vi "DAQmx Create Channel (Power).vi"(0 "task in":refnum<k21>, 1 "voltage setpoint":dbl, 2 "current setpoint":dbl=0.03, 5 "physical channels":tag, 7 "name to assign":string, 9 "output enable":bool=TRUE, 11 "error in":errorcluster) -> (4 "task out":refnum<k21>, 15 "error out":errorcluster)   [LabVIEW 2024]
doc: "Creates channel(s) to source and measure power."
uses:
  nilvaiu.dll
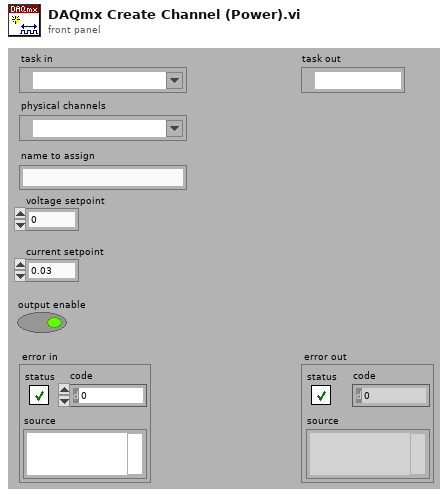
[diagram p1: front panel]
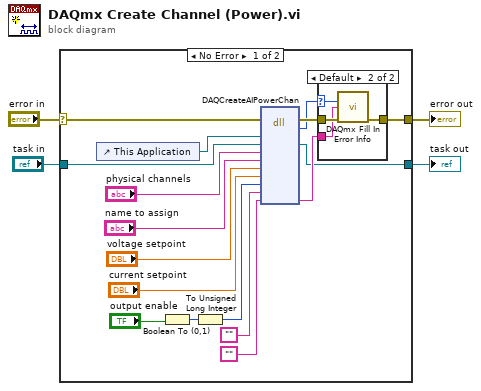
[diagram p0: block diagram]
diagram:
  n1 = case shown="No Error" "error in" {
    selector: "error in" -> [w17 w28]
    tunnel: [w16 w28] -> w4
    tunnel: [w15 w27] -> w3
    tunnel: "task in" -> [w14 w27]
    frame No Error {
      n2 = control-ref of="This Application"() -> (w18:refnum<vi>)
      n3 = Boolean To (0,1)(Boolean="output enable") -> (0, 1=w7:i16)
      n4 = To Unsigned Long Integer(number=w7) -> (unsigned 32bit integer=w5:u32)
      n5 = dll-call lib="nilvaiu.*" fn="DAQCreateAIPowerChan"(error in=w17, "lvAppRef"=w18, "refObjPtr"=w14, "physicalChannelName"="physical channels", "channelNameIn"="name to assign", "voltageSetpoint"="voltage setpoint", "currentSetpoint"="current setpoint", "OutputEnable"=w5, "channelNamesOut"="", "extendedErrorInfo"="") -> (error out=w21:errorcluster, "return type"=w20:i32, "refObjPtr"=w15:refnum<k21>, "extendedErrorInfo"=w19:string)  [unwired: 9 in, 1 out]
      n6 = case shown="Default" w20 {
        selector: w20 -> [_ w24]
        tunnel: w21 -> [w22 w26]
        tunnel: [w22 w25] -> w16
        tunnel: w19 -> [_ w23]
        frame 0 {
        }
        frame Default {
          n7 = call "DAQmx Fill In Error Info.vi"("status code"=w24, "extended error info"=w23, "error in"=w26) -> ("error out"=w25:errorcluster)  [unwired: 1 in, 11 out]
        }
      }
    }
    frame Error {
    }
  }
  "error out" <- w4
  "task out" <- w3
